vi "FilterORT.vi"() -> ()   [LabVIEW 2016]
uses:
  controls/Enum.ctl
  <vilib>/Utility/error.llb/Error Cluster From Error Code.vi
  <vilib>/rvi/errors/niLvFpgaAdjustHostInterfaceError.vi
  <vilib>/rvi/interface/nirviReadWriteControl/nirviReadWriteControl.xnode
  controls/FPGAVIreferenceTypeDef.ctl
  FPGA Bitfiles/qnmController797_usbRIO_controllerFPGAmu.lvbitx
  NiFpgaLv.dll
panel:
  in  "ort.p.fcAvg":i8
  in  "ort.p.fcAvgEnable":bool
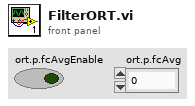
[diagram p1: front panel]
types:
  T1 = typedef "Enum.ctl" = enum16{"Init", "Read", "Write"}
  T2 = typedef "FPGAVIreferenceTypeDef.ctl" = refnum<k20>
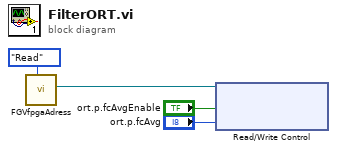
[diagram p0: block diagram]
diagram:
  n1 = call "FGVfpgaAdress.vi"("Enum"=Enum."Read") -> ("FPGA VI Reference Out"=w4:T2)  [unwired: 5 in, 5 out]
  n2 = xnode "Read/Write Control"("FPGA VI Reference In"=w4, "ort.p.fcAvgEnable"="ort.p.fcAvgEnable", "ort.p.fcAvg"="ort.p.fcAvg") -> ()  [unwired: 1 in, 2 out]
